vi "GrowableFunction.vi"(8 "error in":errorcluster, 11 "reference":refnum<vi>) -> (0 "error out":errorcluster, 3 "Function out":refnum<class "GrowableFunction.lvclass">)   [LabVIEW 2014, in "Raspberry Pi Compatible Compiler for LabVIEW.lvlib" / "GrowableFunction.lvclass"]
uses:
  GrowableFunction.lvclass
  NamedBundler/NamedBundler.lvclass
  NamedUnbundler/NamedUnbundler.lvclass
  CompoundArithmetic/CompoundArithmetic.lvclass
  IndexArray/IndexArray.lvclass
  Node/Node.lvclass
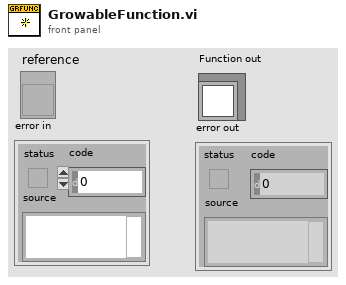
[diagram p1: front panel]
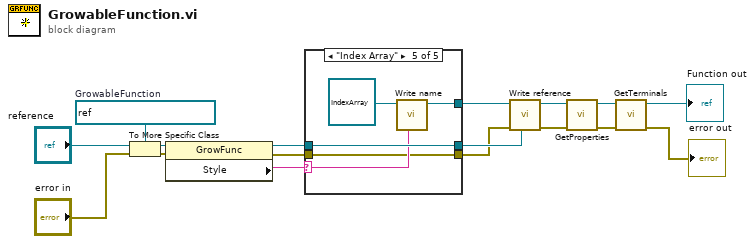
[diagram p0: block diagram]
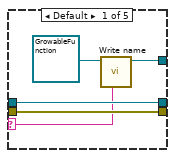
[diagram p2: hidden frame]
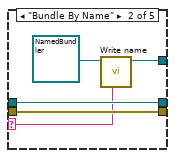
[diagram p3: hidden frame]
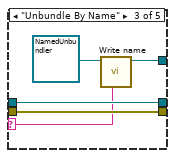
[diagram p4: hidden frame]
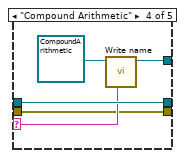
[diagram p5: hidden frame]
diagram:
  w17 = refnum<vi> refnum  # GrowableFunction
  n1 = To More Specific Class(target class=w17, reference="reference", error in="error in") -> (specific class reference=w14:refnum<vi>, error out=w13:errorcluster)
  n2 = property class="GrowFunc"(reference=w14, error in=w13) -> (reference out=w11:refnum<vi>, error out=w8:errorcluster, "Style"=w12:string)
  n3 = case shown="\"Index Array\"" w12 {
    selector: w12 -> [w18 w23 w28 w35 w40]
    tunnel: [w20 w25 w30 w34 w39] -> w10
    tunnel: w11 -> [w22 w27 w32 w37 w42]
    tunnel: [w22 w27 w32 w37 w42] -> w9
    tunnel: w8 -> [w21 w26 w31 w33 w38]
    tunnel: [w21 w26 w31 w33 w38] -> w7
    frame Default {
      n4 = call-dynamic "Write name.vi"("name"=w18, "Node in"=refnum<class "GrowableFunction.lvclass"> refnum ("Function in")) -> ("Node out"=w20:refnum<class "GrowableFunction.lvclass">)  [unwired: 7 in]
    }
    frame "Bundle By Name" {
      n5 = call-dynamic "Write name.vi"("name"=w23, "Node in"=refnum<class "NamedBundler.lvclass"> refnum ("Function in")) -> ("Node out"=w25:refnum<class "NamedBundler.lvclass">)  [unwired: 7 in]
    }
    frame "Unbundle By Name" {
      n6 = call-dynamic "Write name.vi"("name"=w28, "Node in"=refnum<class "NamedUnbundler.lvclass"> refnum ("Function in")) -> ("Node out"=w30:refnum<class "NamedUnbundler.lvclass">)  [unwired: 7 in]
    }
    frame "Compound Arithmetic" {
      n7 = call-dynamic "Write name.vi"("name"=w35, "Node in"=refnum<class "CompoundArithmetic.lvclass"> refnum ("Function in")) -> ("Node out"=w34:refnum<class "CompoundArithmetic.lvclass">)  [unwired: 7 in]
    }
    frame "Index Array" {
      n8 = call-dynamic "Write name.vi"("name"=w40, "Node in"=refnum<class "IndexArray.lvclass"> refnum ("Function in")) -> ("Node out"=w39:refnum<class "IndexArray.lvclass">)  [unwired: 7 in]
    }
  }
  n9 = call-dynamic "Write reference.vi"("reference"=w9, "error in"=w7, "GObject in"=w10) -> ("error out"=w1:errorcluster, "GObject out"=w4:refnum<class "GrowableFunction.lvclass">)  [unwired: 5 in]
  n10 = call-dynamic "GetProperties.vi"("error in"=w1, "GObject in"=w4) -> ("error out"=w2:errorcluster, "GObject out"=w3:refnum<class "GrowableFunction.lvclass">)  [unwired: 8 in]
  n11 = call "GetTerminals.vi"("error in"=w2, "Node in"=w3) -> ("error out"=→"error out":errorcluster, "Node out"=→"Function out":refnum<class "GrowableFunction.lvclass">)  [unwired: 8 in]
